vi "TLB Native Dynamic Events ver 0.05a Local Variable mode.vi"() -> ()   [LabVIEW 2018]
uses:
  Labview Training Phase 2/Enum Controls/States for Action Engine.ctl
  Type def/TLB event states.ctl
  Type def/TLB MHL States.ctl
  <vilib>/Studica/Studica Toolkit/NavX/NavX.lvlib
  <vilib>/Studica/Studica Toolkit/Background/I2C Channel.ctl
  <vilib>/myRIO/Common/Instrument Driver Framework/myRIO v1.0/AI/typedefs/AI Channels Enum.ctl
  <vilib>/myRIO/Common/Instrument Driver Framework/myRIO v1.0/AI/typedefs/AI Channels List.ctl
  <vilib>/Studica/Studica Toolkit/Background/Mxp Selection.ctl
panel:
  out "CM":fxp<+,64,16>
  out "wDistance":dbl
  out "xDistance":dbl
  out "yDistance":dbl
  in  "Reset Encoder 0":bool
  out "Speed":T1
  in  "wTargetSpeed":dbl
  in  "yTargetSpeed":dbl
  in  "xTargetSpeed":dbl
  out "Sharp IR Distance 2":dbl
  out "Sharp IR Distance":dbl
  out "YRPHfH":T2
  out "Displacement":T3
  out "LinearAcceleration":T4
  out "NavX Info Out":T6
  out "Action Queues":string[](array[string])
  out "State logic":T7
  out "Action State":string
  in  "Task condition":bool
  in  "Combo Box":string(combo)
  in  "Stop Queue":bool
  in  "Start Task":bool
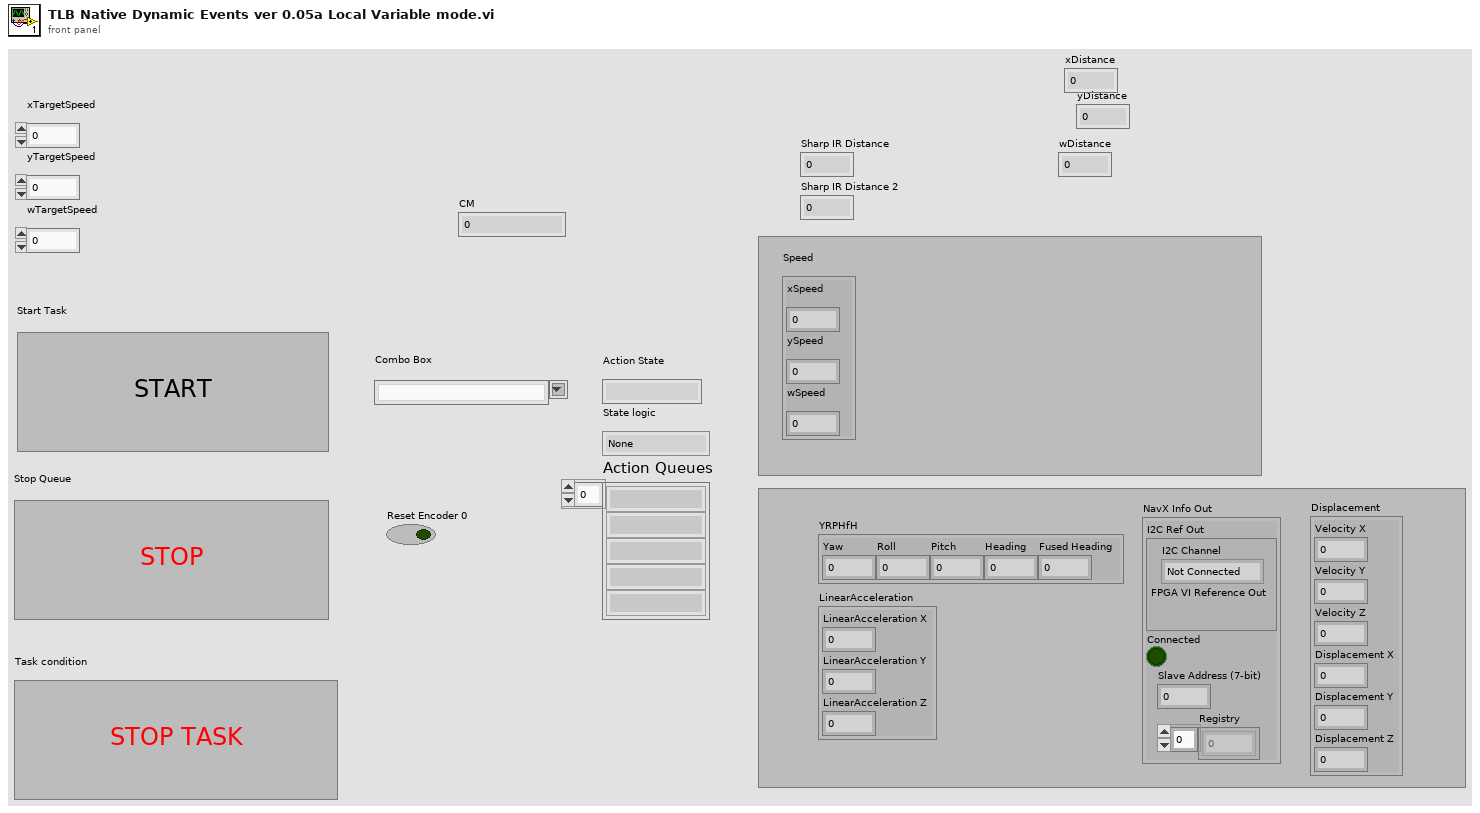
[diagram p1: front panel]
types:
  T1 = cluster{"xSpeed":dbl, "ySpeed":dbl, "wSpeed":dbl}
  T2 = cluster{"Yaw":dbl, "Roll":dbl, "Pitch":dbl, "Heading":dbl, "Fused Heading":dbl}
  T3 = cluster{"Velocity X":dbl, "Velocity Y":dbl, "Velocity Z":dbl, "Displacement X":dbl, "Displacement Y":dbl, "Displacement Z":dbl}
  T4 = cluster{"LinearAcceleration X":dbl, "LinearAcceleration Y":dbl, "LinearAcceleration Z":dbl}
  T5 = typedef "I2C Channel.ctl" = enum16{"Not Connected", "A", "B"}
  T6 = cluster{"I2C Ref Out":cluster{"I2C Channel":T5, "FPGA VI Reference Out":refnum<k20>}, "Connected":bool, "Slave Address (7-bit)":u8, "Registry":u8[]}
  T7 = typedef "TLB MHL States.ctl" = enum16{"None", "Startup", "Idle", "Processing", "Shutdown", "Reset", "Task 1", "Task 2", "Task 3", "Task 4", "Task 4a", "Task 4b", "Task 4c", "Task 4d", "Task 4e", "Task 4f", "Task 4g", "Task 4h", "Acquire image", "Wall follow mode", "Drive Straight"}
  T8 = typedef "States for Action Engine.ctl" = enum16{"Initialize", "Write", "Read"}
  T9 = typedef "TLB event states.ctl" = enum16{"Start Sequence", "Exit", "Start Task 1", "Start Task 2", "Start Task 3", "Start Task 4", "Camera vision", "Wall follow mode", "Idle", "Start Drive Straight"}
  T10 = typedef "Mxp Selection.ctl" = enum16{"MXP A", "MXP B"}
  T11 = typedef "TLB event states.ctl" = enum16{"Start Sequence", "Exit", "Task 1", "Task 2", "Idle"}
  T12 = cluster{"queue out":refnum<queue>, "error out":errorcluster}
  T13 = cluster{"xDistance":dbl, "yDistance":dbl, "wDistance":dbl}
  T14 = typedef "AI Channels List.ctl" = T15[]
  T15 = typedef "AI Channels Enum.ctl" = enum16{"Not Connected", "AudioIn/Left", "AudioIn/Right", "C/AI0", "C/AI1", "A/AI0", "A/AI1", "A/AI2", "A/AI3", "A/AI4", "A/AI5", "A/AI6", "A/AI7", "B/AI0", "B/AI1", "B/AI2", "B/AI3", "B/AI4", "B/AI5", "B/AI6", "B/AI7", "AI/AI0", "AI/AI1", "AI/AI2", "AI/AI3", "A/AI0 (DIFF)", "A/AI1 (DIFF)", "A/AI2 (DIFF)", "A/AI3 (DIFF)", "B/AI0 (DIFF)", "B/AI1 (DIFF)", "B/AI2 (DIFF)", "B/AI3 (DIFF)"}
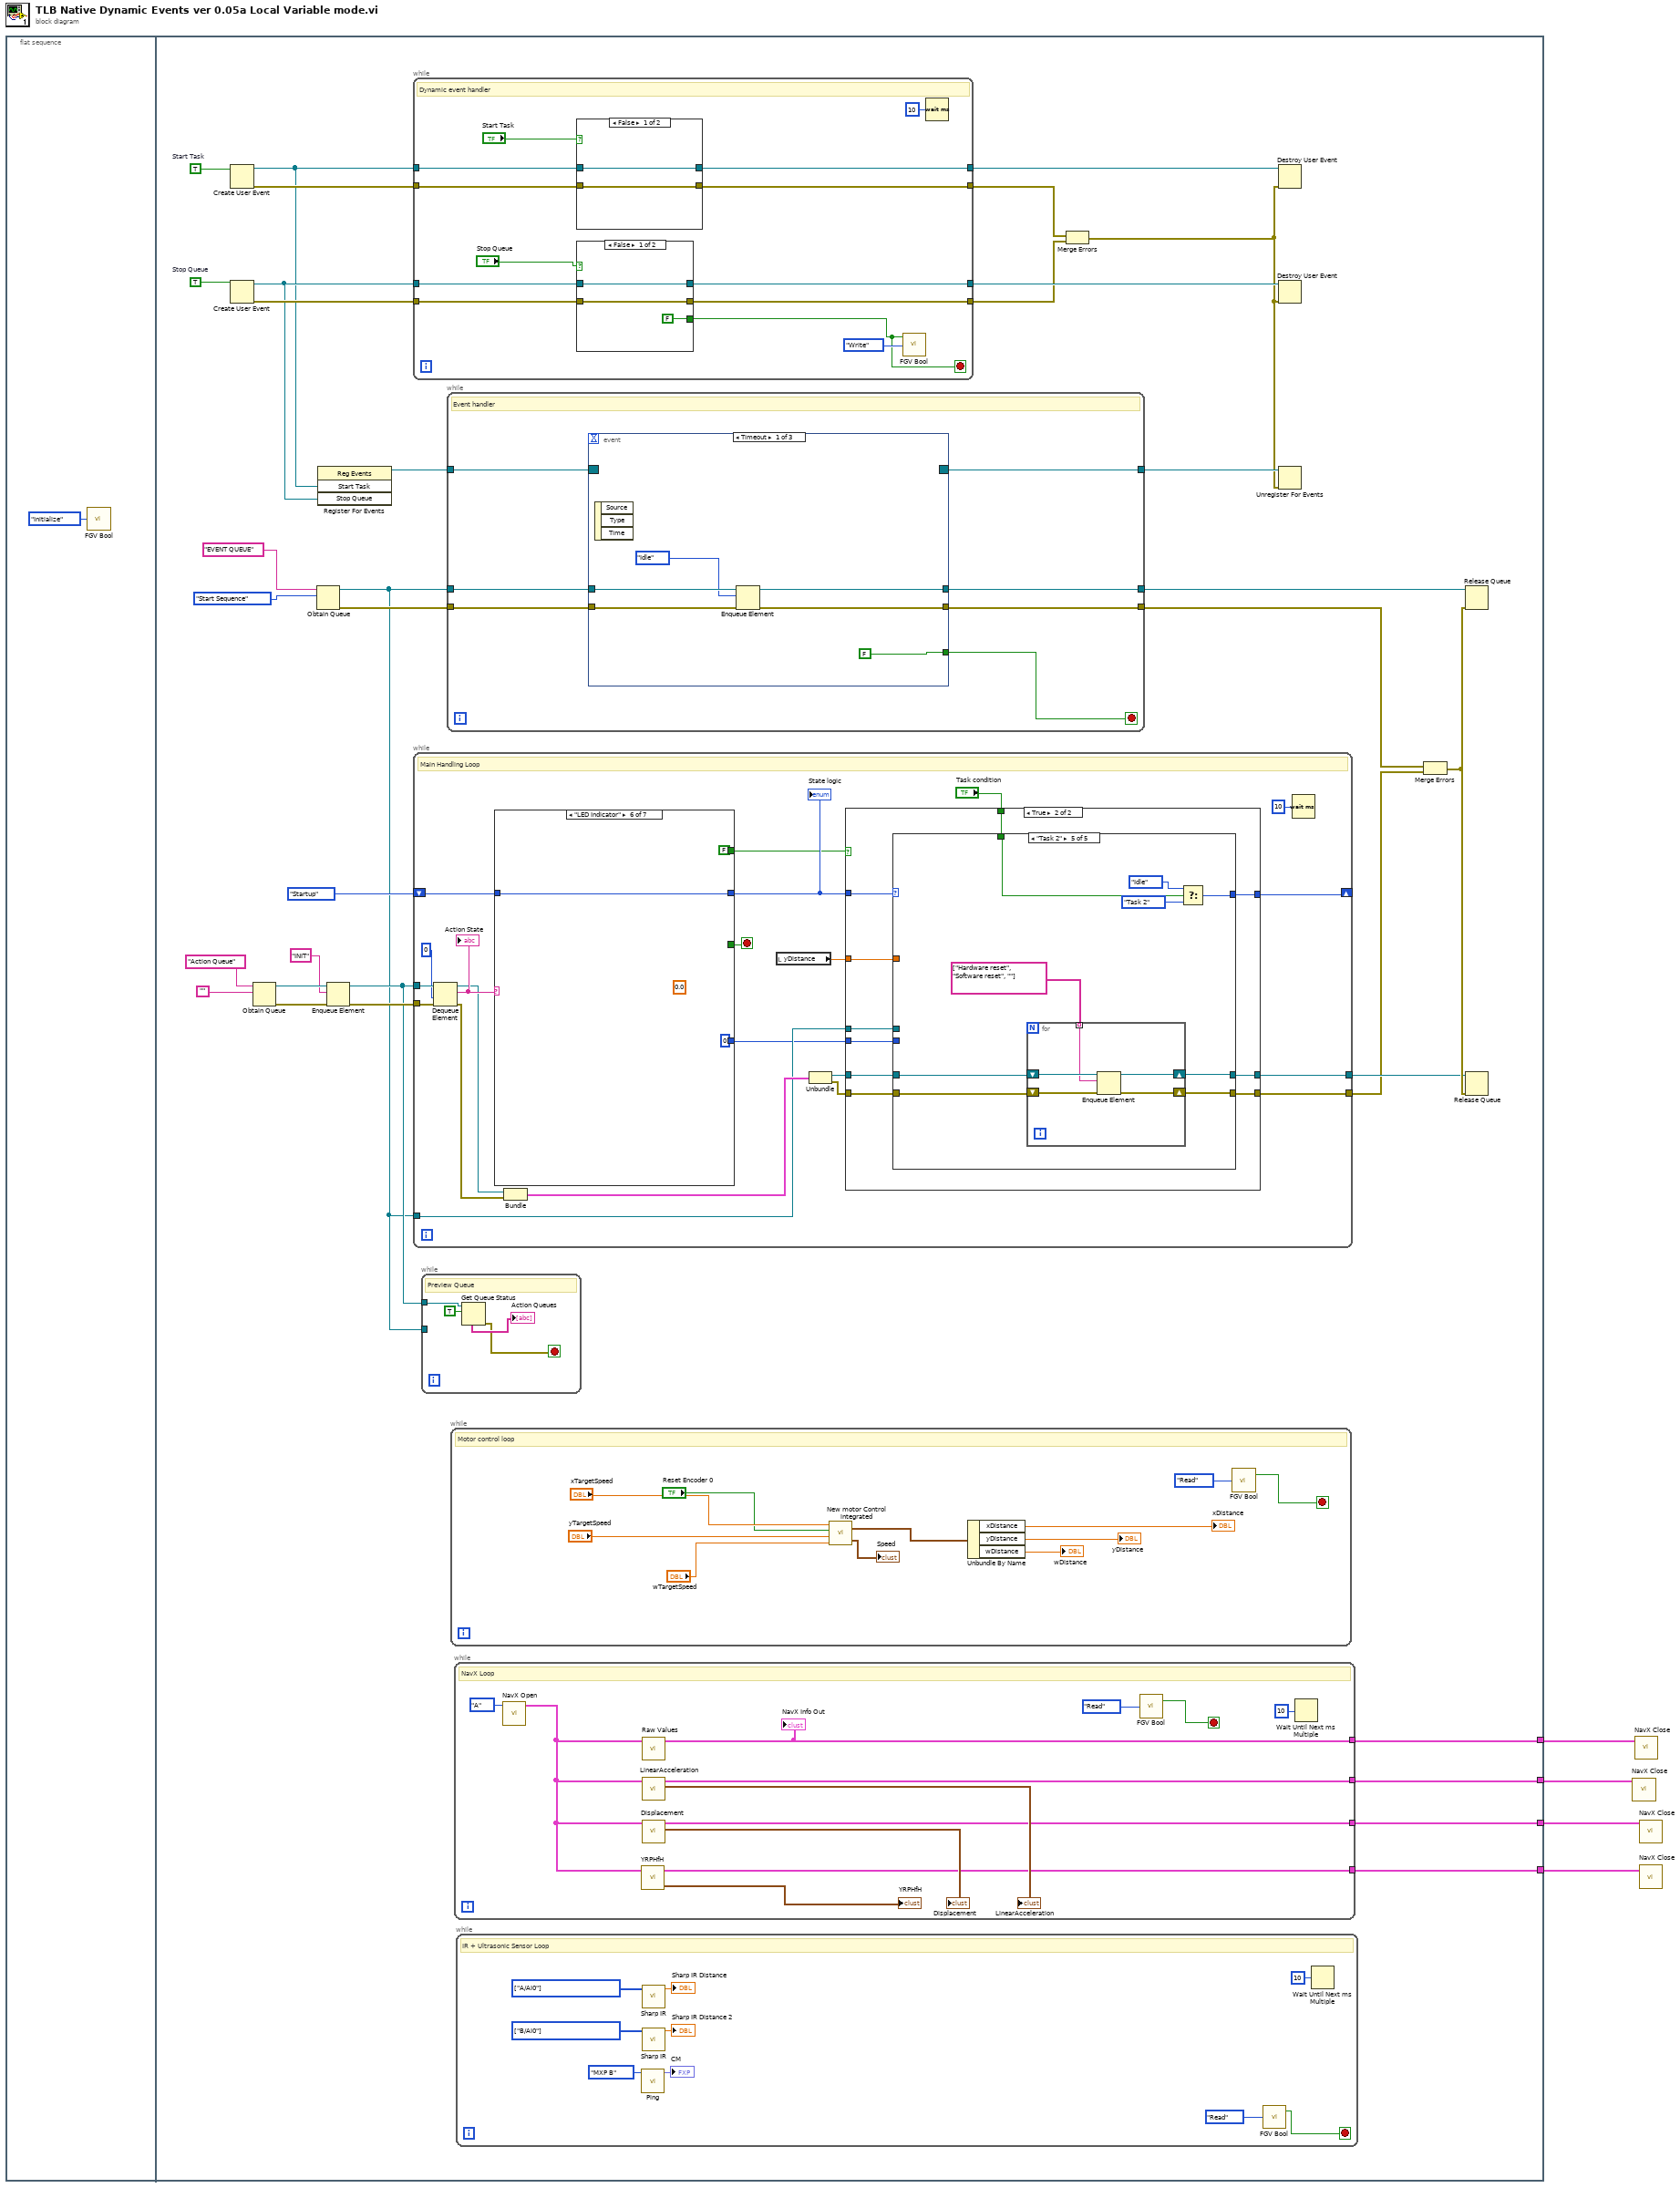
[diagram p0: block diagram]
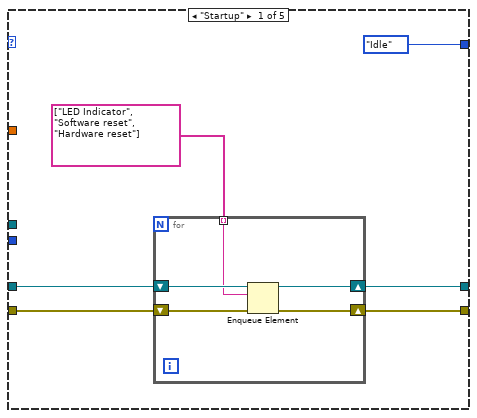
[diagram p3: hidden frame]
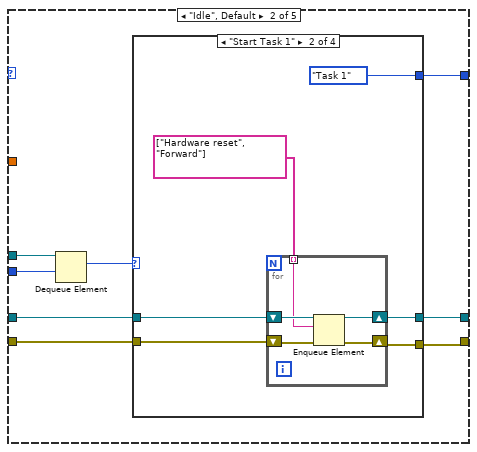
[diagram p4: hidden frame]
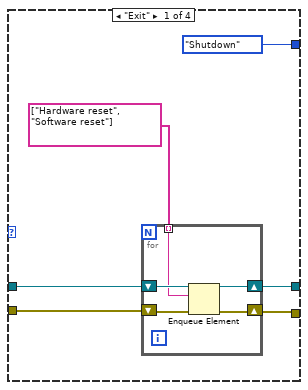
[diagram p5: hidden frame]
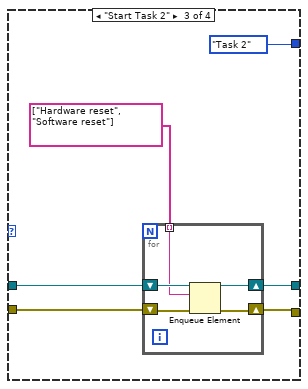
[diagram p6: hidden frame]
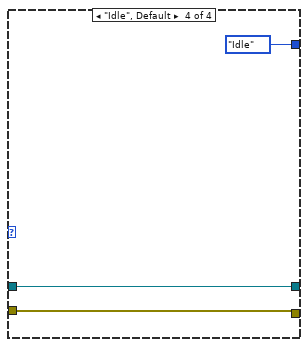
[diagram p7: hidden frame]
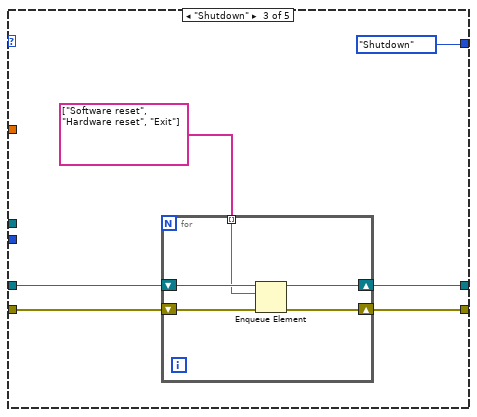
[diagram p8: hidden frame]
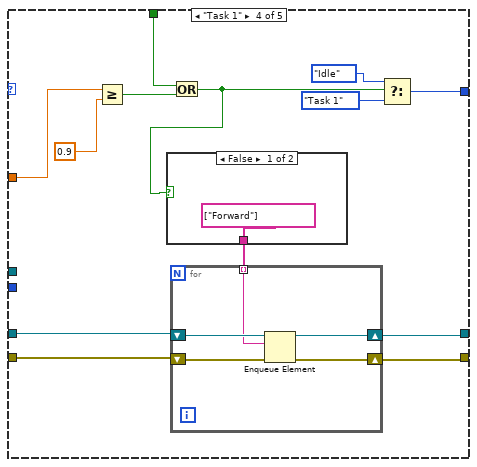
[diagram p9: hidden frame]
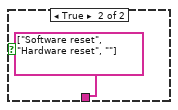
[diagram p10: hidden frame]
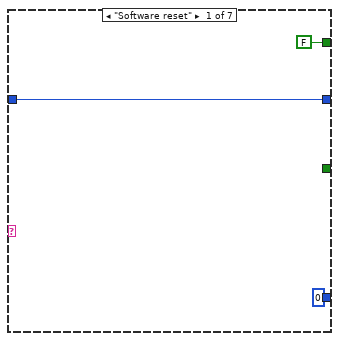
[diagram p11: hidden frame]
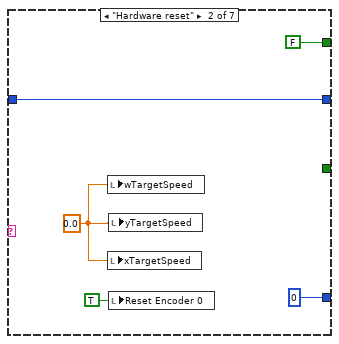
[diagram p12: hidden frame]
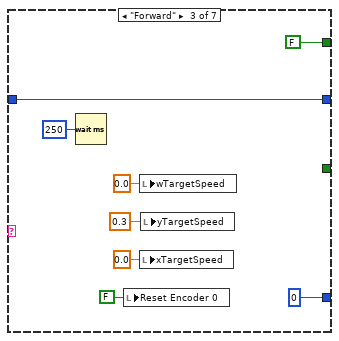
[diagram p13: hidden frame]
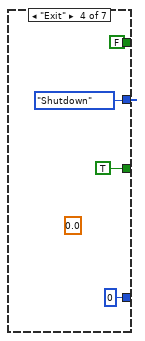
[diagram p14: hidden frame]
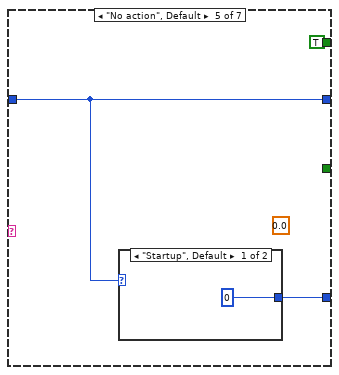
[diagram p15: hidden frame]
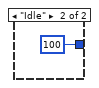
[diagram p16: hidden frame]
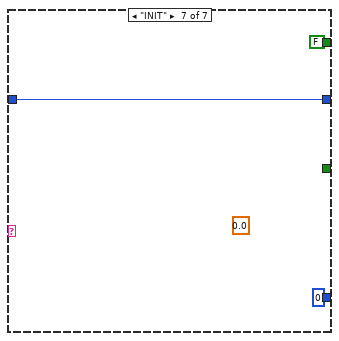
[diagram p17: hidden frame]
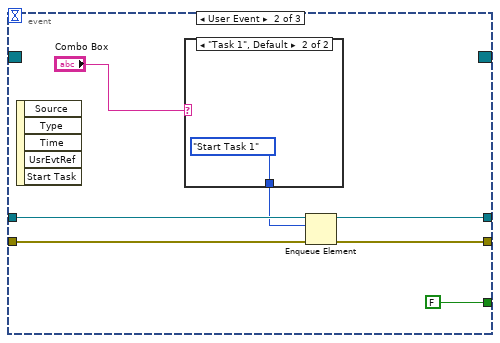
[diagram p18: hidden frame]
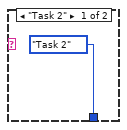
[diagram p19: hidden frame]
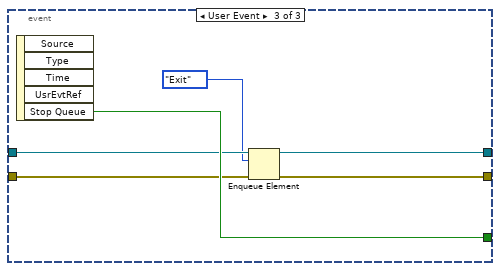
[diagram p20: hidden frame]
diagram:
  n1 = flat-sequence {
    tunnel: [w9] -> w4
    tunnel: [w8] -> w3
    tunnel: [w7] -> w2
    tunnel: [w6] -> w1
    frame #0 {
      n2 = call "FGV Bool.vi"("Init/Read/Write State"=States_for_Action_Engine."Initialize") -> ()  [unwired: 2 in, 2 out]
    }
    frame #1 {
      w39 = TRUE  # Stop Queue
      w38 = TRUE  # Start Task
      n3 = Create User Event(user event datatype=w38) -> (user event=w30:refnum<user-event>, error out=w35:errorcluster)  [unwired: 1 in]
      n4 = Create User Event(user event datatype=w39) -> (user event=w31:refnum<user-event>, error out=w34:errorcluster)  [unwired: 1 in]
      n5 = Obtain Queue(name (unnamed)="Action Queue", element data type="") -> (queue out=w23:refnum<queue>, error out=w19:errorcluster)  [unwired: 3 in, 1 out]
      n6 = Obtain Queue(name (unnamed)="EVENT QUEUE", element data type=TLB_event_states."Start Sequence" ("Enum")) -> (queue out=w10:refnum<queue>, error out=w20:errorcluster)  [unwired: 3 in, 1 out]
      n7 = register-events(w30, w31) -> (reference out=w29:refnum<event-registration>)  [unwired: 2 in, 1 out]
      n8 = Enqueue Element(queue=w23, element="INIT", error in (no error)=w19) -> (queue out=w11:refnum<queue>, error out=w18:errorcluster)  [unwired: 1 in, 1 out]
      n9 = while {
        tunnel: w30 -> [w280]
        tunnel: w31 -> [w279]
        tunnel: [w278] -> w37
        tunnel: [w277] -> w36
        tunnel: w35 -> [w276]
        tunnel: [w275] -> w33
        tunnel: w34 -> [w274]
        tunnel: [w273] -> w32
        stop <- w269 stop-if-true
        # "Dynamic event handler"
        n10 = case shown="False" "Start Task" {
          selector: "Start Task" -> [_ w292]
          tunnel: w280 -> [w291 w296]
          tunnel: [w291 w295] -> w277
          tunnel: w276 -> [w290 w294]
          tunnel: [w290 w293] -> w275
          frame False {
          }
          frame True {
            n11 = Generate User Event(user event=w296, event data cluster=w292, error in=w294) -> (user event out=w295:refnum<user-event>, error out=w293:errorcluster)  [unwired: 1 in]
          }
        }
        n12 = case shown="False" "Stop Queue" {
          selector: "Stop Queue" -> [_ w285]
          tunnel: w279 -> [w284 w289]
          tunnel: [w284 w288] -> w278
          tunnel: w274 -> [w283 w287]
          tunnel: [w283 w286] -> w273
          tunnel: [FALSE w285] -> w269
          frame False {
          }
          frame True {
            n13 = Generate User Event(user event=w289, event data cluster=w285, error in=w287) -> (user event out=w288:refnum<user-event>, error out=w286:errorcluster)  [unwired: 1 in]
          }
        }
        n14 = call "FGV Bool.vi"("Init/Read/Write State"=States_for_Action_Engine."Write", "Input Node"=w269) -> ()  [unwired: 1 in, 2 out]
        n15 = Wait (ms)(milliseconds to wait=u32 10) -> ()  [unwired: 1 out]
      }
      n16 = while {
        tunnel: w10 -> [w82]
        shift-right: [w83] -> _
        shift-left: TLB_MHL_States."Startup" ("Enum") -> [w95]
        tunnel: w11 -> [w93]
        tunnel: w18 -> [w91]
        tunnel: [w85] -> w15
        tunnel: [w84] -> w14
        stop <- w80 stop-if-true
        # "Main Handling Loop"
        n17 = Dequeue Element(queue=w93, timeout in ms (-1)=0, error in (no error)=w91) -> (queue out=w90:refnum<queue>, element=w92:string, error out=w89:errorcluster)  [unwired: 1 out]
        "Action State" <- w92
        n18 = case shown="\"LED Indicator\"" w92 {
          tunnel: [w212 w217 w224 TLB_MHL_States."Shutdown" ("Enum") w232 w237 w240] -> w94
          tunnel: w95 -> [w212 w217 w224 _ w232 w237 w240]
          tunnel: [0 0 0 0 w231 0 0] -> w81
          tunnel: [_ _ _ TRUE _ _ _] -> w80
          tunnel: [FALSE FALSE FALSE FALSE TRUE FALSE FALSE] -> w78
          frame "Software reset" {
          }
          frame "Hardware reset" {
            w214 = 0.0
            n19 = local write "wTargetSpeed"(w214) -> ()
            n20 = local write "xTargetSpeed"(w214) -> ()
            n21 = local write "yTargetSpeed"(w214) -> ()
            n22 = local write "Reset Encoder 0"(TRUE ("Reset Encoder 0")) -> ()
          }
          frame "Forward" {
            n23 = Wait (ms)(milliseconds to wait=u32 250) -> ()  [unwired: 1 out]
            n24 = local write "Reset Encoder 0"(FALSE ("Reset Encoder 0")) -> ()
            n25 = local write "wTargetSpeed"(0.0 ("wTargetSpeed")) -> ()
            n26 = local write "xTargetSpeed"(0.0 ("xTargetSpeed")) -> ()
            n27 = local write "yTargetSpeed"(0.3 ("yTargetSpeed")) -> ()
          }
          frame "Exit" {
            (unwired) 0.0
          }
          frame "No action", Default {
            (unwired) 0.0
            n28 = case shown="\"Startup\", Default" w232 {
              tunnel: [0 100] -> w231
              frame "Startup", Default {
              }
              frame "Idle" {
              }
            }
          }
          frame "LED Indicator" {
            (unwired) 0.0
          }
          frame "INIT" {
            (unwired) 0.0
          }
        }
        "State logic" <- w94
        n29 = Bundle("queue out"=w90, "error out"=w89) -> (w88:T12)  [unwired: 1 in]
        n30 = local read "yDistance"() -> (w76:dbl)
        n31 = Unbundle(w88) -> ("queue out"=w87:refnum<queue>, "error out"=w86:errorcluster)
        n32 = case shown="True" w78 {
          tunnel: w94 -> [w98 w109]
          tunnel: w87 -> [w99 w108]
          tunnel: w86 -> [w97 w107]
          tunnel: [w99 w106] -> w85
          tunnel: [w97 w105] -> w84
          tunnel: [w98 w104] -> w83
          tunnel: w82 -> [_ w103]
          tunnel: w81 -> [_ w102]
          tunnel: "Task condition" -> [_ w101]
          tunnel: w76 -> [_ w100]
          frame False {
          }
          frame True {
            n33 = case shown="\"Task 2\"" w109 {
              tunnel: w108 -> [w115 w122 w168 w183 w198]
              tunnel: w107 -> [w114 w124 w166 w182 w197]
              tunnel: [w113 w125 w167 w185 w200] -> w106
              tunnel: [w112 w123 w165 w184 w199] -> w105
              tunnel: [TLB_MHL_States."Idle" ("Enum") w126 TLB_MHL_States."Shutdown" ("Enum") w186 w202] -> w104
              tunnel: w103 -> [_ w128 _ _ _]
              tunnel: w102 -> [_ w121 _ _ _]
              tunnel: w101 -> [_ _ _ w180 w196]
              tunnel: w100 -> [_ _ _ w177 _]
              frame "Startup" {
                n34 = for {
                  shift-right: [w118] -> w113
                  shift-left: w115 -> [w120]
                  shift-right: [w117] -> w112
                  shift-left: w114 -> [w119]
                  tunnel: string[] ["LED Indicator", "Software reset", "Hardware reset"] -> [w116] mode=indexing
                  n35 = Enqueue Element(queue=w120, element=w116, error in (no error)=w119) -> (queue out=w118:refnum<queue>, error out=w117:errorcluster)  [unwired: 1 in, 1 out]
                }
              }
              frame "Idle", Default {
                n36 = Dequeue Element(queue=w128, timeout in ms (-1)=w121) -> (element=w127:T9)  [unwired: 1 in, 3 out]
                n37 = case shown="\"Start Task 1\"" w127 {
                  tunnel: [TLB_MHL_States."Shutdown" ("Enum") TLB_MHL_States."Task 1" ("Enum") TLB_MHL_States."Task 2" ("Enum") TLB_MHL_States."Idle" ("Enum")] -> w126
                  tunnel: [w131 w144 w153 w163] -> w125
                  tunnel: w122 -> [w133 w143 w155 w163]
                  tunnel: w124 -> [w132 w142 w154 w162]
                  tunnel: [w130 w141 w152 w162] -> w123
                  frame "Exit" {
                    n38 = for {
                      shift-right: [w139] -> w131
                      shift-left: w133 -> [w138]
                      shift-right: [w136] -> w130
                      shift-left: w132 -> [w137]
                      tunnel: string[] ["Hardware reset", "Software reset"] -> [w135] mode=indexing
                      n39 = Enqueue Element(queue=w138, element=w135, error in (no error)=w137) -> (queue out=w139:refnum<queue>, error out=w136:errorcluster)  [unwired: 1 in, 1 out]
                    }
                  }
                  frame "Start Task 1" {
                    n40 = for {
                      shift-right: [w150] -> w144
                      shift-left: w143 -> [w149]
                      shift-right: [w147] -> w141
                      shift-left: w142 -> [w148]
                      tunnel: string[] ["Hardware reset", "Forward"] -> [w146] mode=indexing
                      n41 = Enqueue Element(queue=w149, element=w146, error in (no error)=w148) -> (queue out=w150:refnum<queue>, error out=w147:errorcluster)  [unwired: 1 in, 1 out]
                    }
                  }
                  frame "Start Task 2" {
                    n42 = for {
                      shift-right: [w161] -> w153
                      shift-left: w155 -> [w160]
                      shift-right: [w158] -> w152
                      shift-left: w154 -> [w159]
                      tunnel: string[] ["Hardware reset", "Software reset"] -> [w157] mode=indexing
                      n43 = Enqueue Element(queue=w160, element=w157, error in (no error)=w159) -> (queue out=w161:refnum<queue>, error out=w158:errorcluster)  [unwired: 1 in, 1 out]
                    }
                  }
                  frame "Idle", Default {
                  }
                }
              }
              frame "Shutdown" {
                n44 = for {
                  shift-right: [w173] -> w167
                  shift-left: w168 -> [w175]
                  shift-right: [w172] -> w165
                  shift-left: w166 -> [w174]
                  tunnel: string[] ["Software reset", "Hardware reset", "Exit"] -> [w171] mode=indexing
                  n45 = Enqueue Element(queue=w175, element=w171, error in (no error)=w174) -> (queue out=w173:refnum<queue>, error out=w172:errorcluster)  [unwired: 1 in, 1 out]
                }
              }
              frame "Task 1" {
                n46 = Greater Or Equal?(x=w177, y=0.9 ("x")) -> (x >= y?=w179:bool)
                n47 = Or(x=w180, y=w179) -> (x .or. y?=w178:bool)
                n48 = case shown="False" w178 {
                  tunnel: [string[] ["Forward"] string[] ["Software reset", "Hardware reset", ""]] -> w181
                  frame False {
                  }
                  frame True {
                  }
                }
                n49 = for {
                  shift-right: [w193] -> w185
                  shift-left: w183 -> [w195]
                  shift-right: [w192] -> w184
                  shift-left: w182 -> [w194]
                  tunnel: w181 -> [w191] mode=indexing
                  n50 = Enqueue Element(queue=w195, element=w191, error in (no error)=w194) -> (queue out=w193:refnum<queue>, error out=w192:errorcluster)  [unwired: 1 in, 1 out]
                }
                n51 = Select(t=TLB_MHL_States."Idle" ("Enum"), s=w178, f=TLB_MHL_States."Task 1" ("Enum")) -> (s? t:f=w186:T7)
              }
              frame "Task 2" {
                n52 = for {
                  shift-right: [w207] -> w200
                  shift-left: w198 -> [w209]
                  shift-right: [w206] -> w199
                  shift-left: w197 -> [w208]
                  tunnel: string[] ["Hardware reset", "Software reset", ""] -> [w205] mode=indexing
                  n53 = Enqueue Element(queue=w209, element=w205, error in (no error)=w208) -> (queue out=w207:refnum<queue>, error out=w206:errorcluster)  [unwired: 1 in, 1 out]
                }
                n54 = Select(t=TLB_MHL_States."Idle" ("Enum"), s=w196, f=TLB_MHL_States."Task 2" ("Enum")) -> (s? t:f=w202:T7)
              }
            }
          }
        }
        n55 = Wait (ms)(milliseconds to wait=u32 10) -> ()  [unwired: 1 out]
      }
      n56 = while {
        tunnel: w11 -> [w73]
        tunnel: w10 -> [_]
        stop <- w72 stop-if-true
        # "Preview Queue"
        n57 = Get Queue Status(queue=w73, return elements? (F)=TRUE) -> (error out=w72:errorcluster, elements=→"Action Queues":string[])  [unwired: 1 in, 6 out]
      }
      n58 = while {
        tunnel: w29 -> [w247]
        tunnel: [w246] -> w28
        tunnel: w10 -> [w244]
        tunnel: [w243] -> w27
        tunnel: w20 -> [w242]
        tunnel: [w241] -> w17
        stop <- w245 stop-if-true
        # "Event handler"
        n59 = event shown="[0] Timeout" {
          selector: w247 -> [_ _ _]
          dyn-events: [_ _ _] -> w246
          timeout: _ -> [_ _ _]
          tunnel: [FALSE FALSE w268] -> w245
          tunnel: w244 -> [w252 w259 w266]
          tunnel: [w251 w258 w267] -> w243
          tunnel: w242 -> [w249 w255 w264]
          tunnel: [w248 w254 w263] -> w241
          event Timeout {
            n60 = event-data() -> ()  [unwired: 1 in, 3 out]
            n61 = Enqueue Element(queue=w252, element=TLB_event_states."Idle" ("Enum"), error in (no error)=w249) -> (queue out=w251:refnum<queue>, error out=w248:errorcluster)  [unwired: 1 in, 1 out]
          }
          event User Event {
            n62 = event-data() -> ()  [unwired: 1 in, 5 out]
            n63 = case shown="\"Task 1\", Default" "Combo Box" {
              tunnel: [TLB_event_states."Task 2" ("Enum") TLB_event_states."Start Task 1" ("Enum")] -> w256
              frame "Task 2" {
              }
              frame "Task 1", Default {
              }
            }
            n64 = Enqueue Element(queue=w259, element=w256, error in (no error)=w255) -> (queue out=w258:refnum<queue>, error out=w254:errorcluster)  [unwired: 1 in, 1 out]
          }
          event User Event {
            n65 = event-data() -> ("Stop Queue"=w268:bool)  [unwired: 1 in, 4 out]
            n66 = Enqueue Element(queue=w266, element=TLB_event_states."Exit" ("Enum"), error in (no error)=w264) -> (queue out=w267:refnum<queue>, error out=w263:errorcluster)  [unwired: 1 in, 1 out]
          }
        }
      }
      n67 = while {
        stop <- w70 stop-if-true
        # "Motor control loop"
        n68 = call "New motor Control integrated.vi"("wTargetSpeed"="wTargetSpeed", "yTargetSpeed"="yTargetSpeed", "xTargetSpeed"="Reset Encoder 0", "Reset Encoders"="xTargetSpeed") -> ("Speed"=→"Speed":T1, "Distance"=w64:T13)
        n69 = Unbundle By Name(w64) -> ("xDistance"=→"xDistance":dbl, "yDistance"=→"yDistance":dbl, "wDistance"=→"wDistance":dbl)
        n70 = call "FGV Bool.vi"("Init/Read/Write State"=States_for_Action_Engine."Read") -> ("Output node"=w70:bool)  [unwired: 2 in, 1 out]
      }
      n71 = while {
        tunnel: [w57] -> w9
        tunnel: [w53] -> w8
        tunnel: [w52] -> w7
        tunnel: [w51] -> w6
        stop <- w59 stop-if-true
        # "NavX Loop"
        n72 = call <vilib>:"NavX Open.vi"("I2C Channel"=I2C_Channel."A") -> ("NavX Info"=w49:T6)  [unwired: 9 in, 1 out]
        n73 = call <vilib>:"YRPHfH.vi"("NavX Info In"=w49) -> ("YRPHfH"=→"YRPHfH":T2, "NavX Info Out"=w52:T6)  [unwired: 3 in]
        n74 = call <vilib>:"Raw Values.vi"("NavX Info In"=w49) -> ("NavX Info Out"=w57:T6)  [unwired: 8 in, 1 out]
        "NavX Info Out" <- w57
        n75 = call <vilib>:"LinearAcceleration.vi"("NavX Info In"=w49) -> ("LinearAcceleration"=→"LinearAcceleration":T4, "NavX Info Out"=w53:T6)  [unwired: 9 in]
        n76 = call <vilib>:"Displacement.vi"("NavX Info In"=w49) -> ("Displacement"=→"Displacement":T3, "NavX Info Out"=w51:T6)  [unwired: 9 in]
        n77 = call "FGV Bool.vi"("Init/Read/Write State"=States_for_Action_Engine."Read") -> ("Output node"=w59:bool)  [unwired: 2 in, 1 out]
        n78 = Wait Until Next ms Multiple(millisecond multiple=u32 10) -> ()  [unwired: 1 out]
      }
      n79 = while {
        stop <- w42 stop-if-true
        w47 = T14 [enum."B/AI0"] items=["Not Connected", "AudioIn/Left", "AudioIn/Right", "C/AI0", "C/AI1", "A/AI0", "A/AI1", "A/AI2", "A/AI3", "A/AI4", "A/AI5", "A/AI6", "A/AI7", "B/AI0", "B/AI1", "B/AI2", "B/AI3", "B/AI4", "B/AI5", "B/AI6", "B/AI7", "AI/AI0", "AI/AI1", "AI/AI2", "AI/AI3", "A/AI0 (DIFF)", "A/AI1 (DIFF)", "A/AI2 (DIFF)", "A/AI3 (DIFF)", "B/AI0 (DIFF)", "B/AI1 (DIFF)", "B/AI2 (DIFF)", "B/AI3 (DIFF)"] ("AI Channel")
        w48 = T14 [enum."A/AI0"] items=["Not Connected", "AudioIn/Left", "AudioIn/Right", "C/AI0", "C/AI1", "A/AI0", "A/AI1", "A/AI2", "A/AI3", "A/AI4", "A/AI5", "A/AI6", "A/AI7", "B/AI0", "B/AI1", "B/AI2", "B/AI3", "B/AI4", "B/AI5", "B/AI6", "B/AI7", "AI/AI0", "AI/AI1", "AI/AI2", "AI/AI3", "A/AI0 (DIFF)", "A/AI1 (DIFF)", "A/AI2 (DIFF)", "A/AI3 (DIFF)", "B/AI0 (DIFF)", "B/AI1 (DIFF)", "B/AI2 (DIFF)", "B/AI3 (DIFF)"] ("AI Channel")
        # "IR + Ultrasonic Sensor Loop"
        n80 = call <vilib>:"Ping.vi"("Mxp Side"=Mxp_Selection."MXP B") -> ("CM"=→"CM":fxp<+,64,16>)  [unwired: 8 in, 2 out]
        n81 = call <vilib>:"Sharp IR.vi"("AI Channel"=w48) -> ("Sharp IR Distance"=→"Sharp IR Distance":dbl)  [unwired: 8 in, 2 out]
        n82 = call <vilib>:"Sharp IR.vi"("AI Channel"=w47) -> ("Sharp IR Distance"=→"Sharp IR Distance 2":dbl)  [unwired: 8 in, 2 out]
        n83 = call "FGV Bool.vi"("Init/Read/Write State"=States_for_Action_Engine."Read") -> ("Output node"=w42:bool)  [unwired: 2 in, 1 out]
        n84 = Wait Until Next ms Multiple(millisecond multiple=u32 10) -> ()  [unwired: 1 out]
      }
      n85 = Merge Errors(w33, w32) -> (w13:errorcluster)
      n86 = Destroy User Event(user event=w36, error in=w13) -> ()  [unwired: 1 out]
      n87 = Destroy User Event(user event=w37, error in=w13) -> ()  [unwired: 1 out]
      n88 = Unregister For Events(event registration refnum=w28, error in=w13) -> ()  [unwired: 1 out]
      n89 = Merge Errors(w17, w14) -> (w16:errorcluster)
      n90 = Release Queue(queue=w27, error in (no error)=w16) -> ()  [unwired: 1 in, 3 out]
      n91 = Release Queue(queue=w15, error in (no error)=w16) -> ()  [unwired: 1 in, 3 out]
    }
  }
  n92 = call <vilib>:"NavX Close.vi"("NavX Info In"=w3) -> ()  [unwired: 10 in, 1 out]
  n93 = call <vilib>:"NavX Close.vi"("NavX Info In"=w4) -> ()  [unwired: 10 in, 1 out]
  n94 = call <vilib>:"NavX Close.vi"("NavX Info In"=w1) -> ()  [unwired: 10 in, 1 out]
  n95 = call <vilib>:"NavX Close.vi"("NavX Info In"=w2) -> ()  [unwired: 10 in, 1 out]
